vi "test_plot.vi"() -> ()   [LabVIEW 2021]
panel:
  in  "p":dbl[](array[numeric])=[1.0, 1.0, 1.0, 3.0]
  in  "start":i32=-3
  in  "end":i32=3
  in  "N":i32=200
  out "XY Graph":cluster{dbl[], "f(X;p)":dbl[]}(graph)
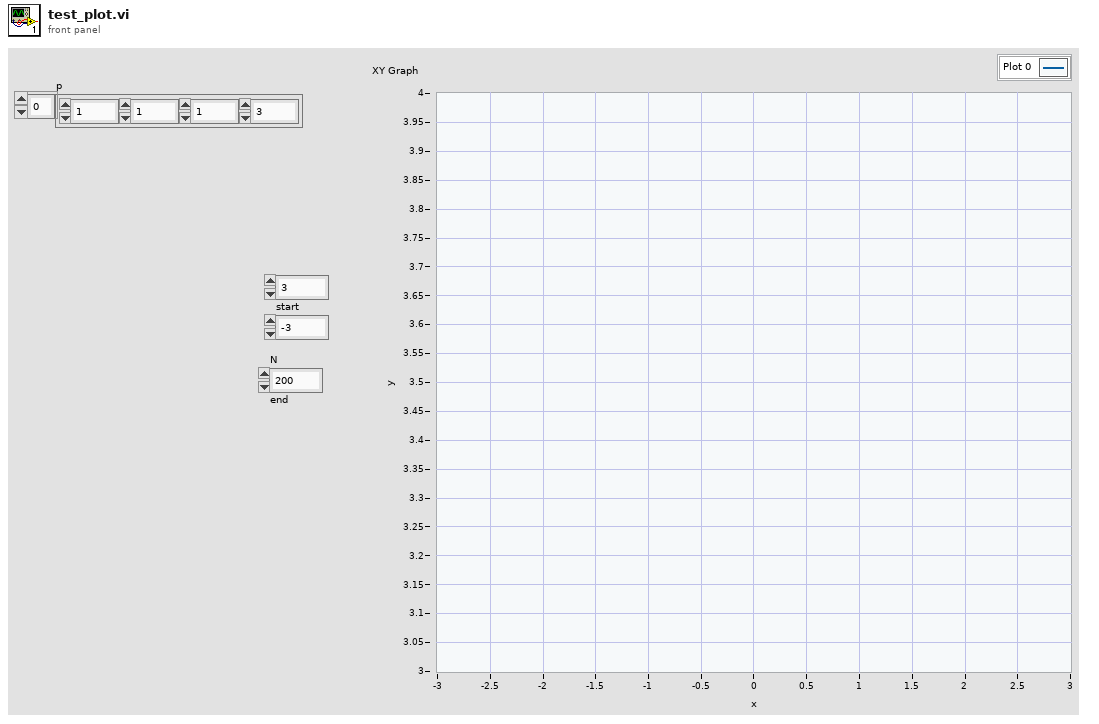
[diagram p1: front panel]
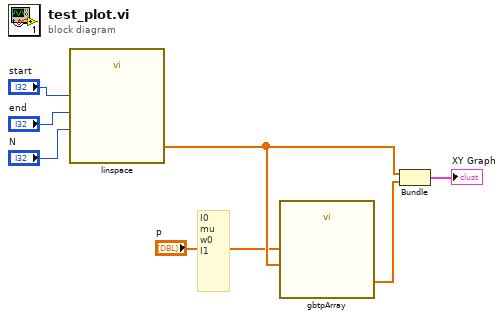
[diagram p0: block diagram]
diagram:
  # "I0\nmu\nw0\nI1"
  n1 = call "linspace.vi"("N"="N", "end"="end", "start"="start") -> ("X"=w2:dbl[])
  n2 = call "gbtpArray.vi"("X"=w2, "P"="p") -> ("f(X;P)"=w3:dbl[])
  n3 = Bundle("X"=w2, "f(X;P)"=w3) -> (→"XY Graph":cluster{"X":dbl[], "f(X;P)":dbl[]})  [unwired: 1 in]
